vi "Write Index of Plugin.vi"(8 "error in (no error)":errorcluster, 10 "Index of Plugin":i32, 11 "Plugin Handler Launch Plugin in":refnum<class "Plugin Handler Launch Plugin.lvclass">) -> (0 "error out":errorcluster, 3 "Plugin Handler Launch Plugin out":refnum<class "Plugin Handler Launch Plugin.lvclass">)   [LabVIEW 2011, in "Plugin Handler Launch Plugin.lvclass"]
uses:
  Plugin Handler Launch Plugin.lvclass
  Plugin Handler Launch Plugin.lvclass/Plugin Handler Launch Plugin.ctl
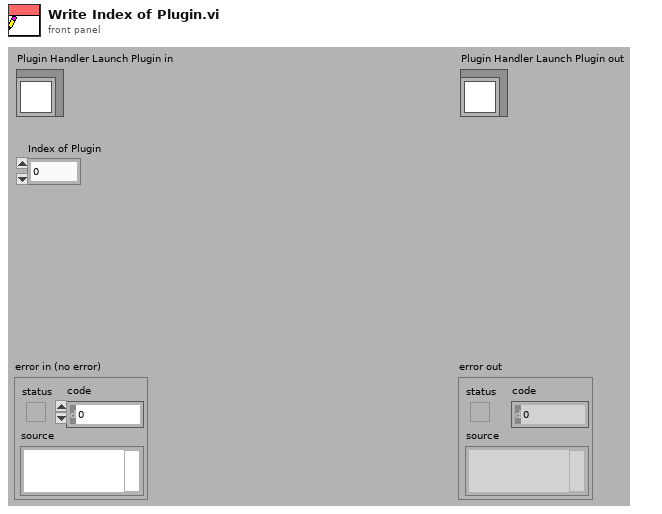
[diagram p1: front panel]
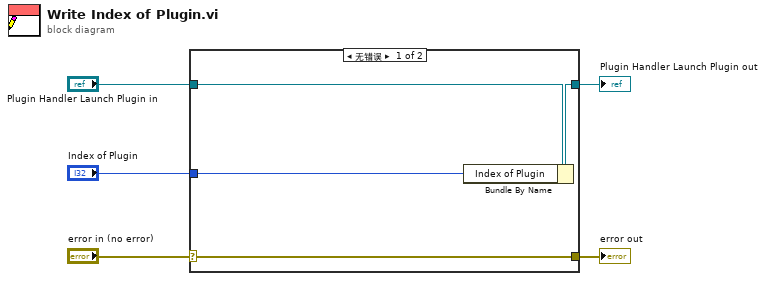
[diagram p0: block diagram]
diagram:
  n1 = case shown="无错误" "error in (no error)" {
    selector: "error in (no error)" -> [w9 w10]
    tunnel: [w9 w10] -> w4
    tunnel: [w7 w11] -> w2
    tunnel: "Plugin Handler Launch Plugin in" -> [w8 w11]
    tunnel: "Index of Plugin" -> [w6 _]
    frame No Error {
      n2 = Bundle By Name(cluster=w8, "Index of Plugin"=w6) -> (w7:refnum<class "Plugin Handler Launch Plugin.lvclass">)
    }
    frame Error {
    }
  }
  "error out" <- w4
  "Plugin Handler Launch Plugin out" <- w2
